vi "SCC File Properties.vi"(8 "error in (no error)":errorcluster, 10 "file path":path, 11 "source control reference in":T1) -> (0 "error out":errorcluster, 2 "status message":string, 3 "source control reference out":T1, 5 "file changed?":bool)   [LabVIEW 2017, in "NI_SCC.lvlib"]
doc: "Displays a dialog box that contains the source control properties of a specified file, such as the file type and revision number. Some source control providers also return properties in the <B>status message</B> output."
uses:
  <vilib>/SourceControl/sccapi/NI_SCC.lvlib
  <vilib>/SourceControl/sccapi/SCCAPI Refnum.ctl
  <vilib>/SourceControl/sccapi/SCCAPI SCC Operations.ctl
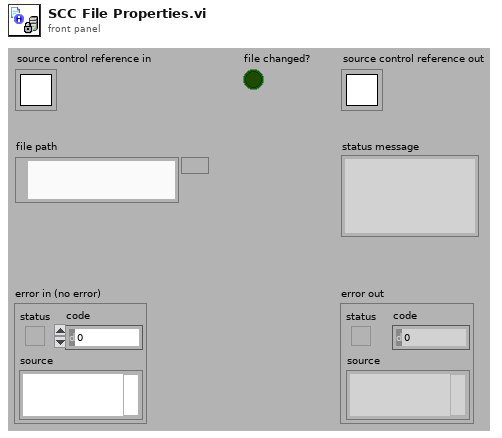
[diagram p1: front panel]
types:
  T1 = typedef "NI_SCC.lvlib/SCCAPI Refnum.ctl" = refnum<k1>
  T2 = typedef "NI_SCC.lvlib/SCCAPI SCC Operations.ctl" = enum16{"Add", "Check In", "Check Out", "Close Project", "Compare Files", "Compare VIs", "Configure Project", "File History", "File Properties", "File Status", "Find All Providers", "Get Advanced Command Options", "Get File Copy", "Get Latest Version", "Get Project Name", "Get StaticVI Path", "Initialize", "Not A Source Control Reference", "Open Project", "Provider Supports Functionality", "Remove", "Run Provider", "Undo Check Out", "Uninitialize", "Is File In Local Path"}
  T3 = typedef "SCCAPI Refnum.ctl" = refnum<k1>
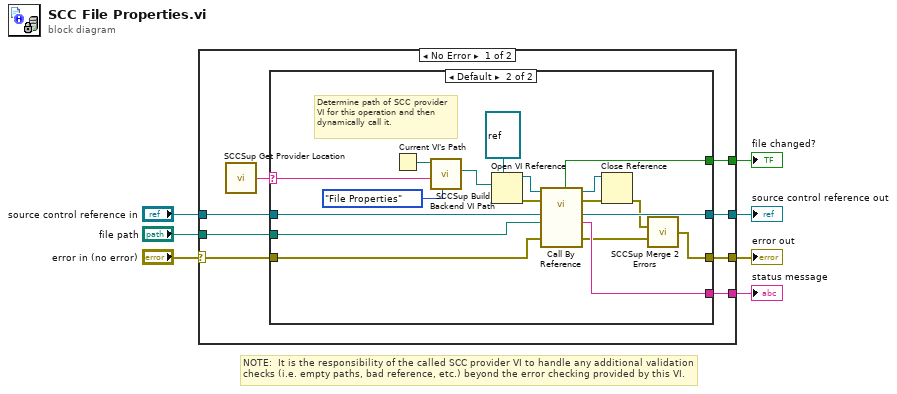
[diagram p0: block diagram]
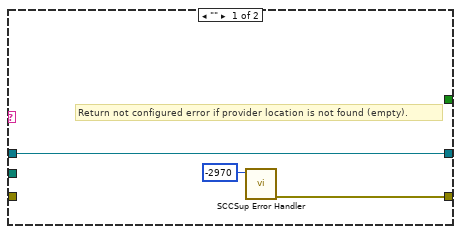
[diagram p2: hidden frame]
diagram:
  # "NOTE:  It is the responsibility of the called SCC provider VI to handle any additional validation checks (i.e. empty paths, bad reference, etc.) beyond the error checking provided by this VI."
  n1 = case shown="No Error" "error in (no error)" {
    selector: "error in (no error)" -> [w9 w38]
    tunnel: [w15 w38] -> w6
    tunnel: "source control reference in" -> [w14 w37]
    tunnel: [w13 _] -> w4
    tunnel: [w12 w37] -> w3
    tunnel: "file path" -> [w11 _]
    tunnel: [w8 _] -> w1
    frame No Error {
      n2 = call <vilib>:"SCCSup Get Provider Location.vi"() -> ("provider location"=w10:string)  [unwired: 6 in]
      n3 = case shown="Default" w10 {
        selector: w10 -> [_ w21]
        tunnel: [w16 w36] -> w15
        tunnel: w14 -> [w18 w28]
        tunnel: [_ w35] -> w13
        tunnel: [w18 w29] -> w12
        tunnel: w11 -> [_ w27]
        tunnel: w9 -> [_ w20]
        tunnel: [_ w19] -> w8
        frame "" {
          # "Return not configured error if provider location is not found (empty)."
          n4 = call <vilib>:"SCCSup Error Handler.vi"("scc error code"=-2970 ("code")) -> ("error out"=w16:errorcluster)  [unwired: 10 in]
        }
        frame Default {
          # "Determine path of SCC provider VI for this operation and then dynamically call it."
          n5 = Current VI's Path() -> (path=w23:path)
          n6 = call <vilib>:"SCCSup Build Backend VI Path.vi"("scc operation"=SCCAPI_SCC_Operations."File Properties", "provider location"=w21, "caller path"=w23) -> ("scc backend VI path"=w24:path)  [unwired: 8 in]
          n7 = Open VI Reference(type specifier VI Refnum (for type only)=refnum<vi> refnum, vi path=w24) -> (vi reference=w33:refnum<vi>, error out=w32:errorcluster)  [unwired: 4 in]
          n8 = call-by-ref "?"(reference=w33, error in=w32, "error in (no error)"=w20, "filename"=w27, "source control reference in"=w28) -> (reference out=w31:refnum<vi>, error out=w30:errorcluster, 0:"error out"=w25:errorcluster, "status message"=w35:string, "source control reference out"=w29:T3, "file changed?"=w19:bool)  [unwired: 5 in]
          n9 = Close Reference(reference=w31, error in (no error)=w30) -> (error out=w26:errorcluster)
          n10 = call <vilib>:"SCCSup Merge 2 Errors.vi"("Error IO 1"=w26, "Error IO 2"=w25) -> ("Error IO out"=w36:errorcluster)  [unwired: 13 in]
        }
      }
    }
    frame Error {
    }
  }
  "error out" <- w6
  "status message" <- w4
  "source control reference out" <- w3
  "file changed?" <- w1
